vi "NumIntegrate_Rkf45_Ax_Bu_K.vi"(5 "A":T1, 6 "MaxError":dbl=1e-06, 7 "B":T1, 8 "dT_Seconds":dbl, 9 "K":T1, 10 "U":T1, 11 "X":T1) -> (1 "IterationCount":i32, 3 "Return X":T1)   [LabVIEW 2019, in "Trajectory_Library.lvlib"]
doc: "Creates a new LINEAR SYSTEM data cluster with the specified values. \n\n\nInputs: \n - XXX -- XXX.\n\nOutputs:\n - XXX -- XXX."
uses:
  Trajectory_Library.lvlib
  <vilib>/Analysis/Matrix/Datatypes/RealMatrix.ctl
  <vilib>/Analysis/Matrix/NI_Matrix.lvlib
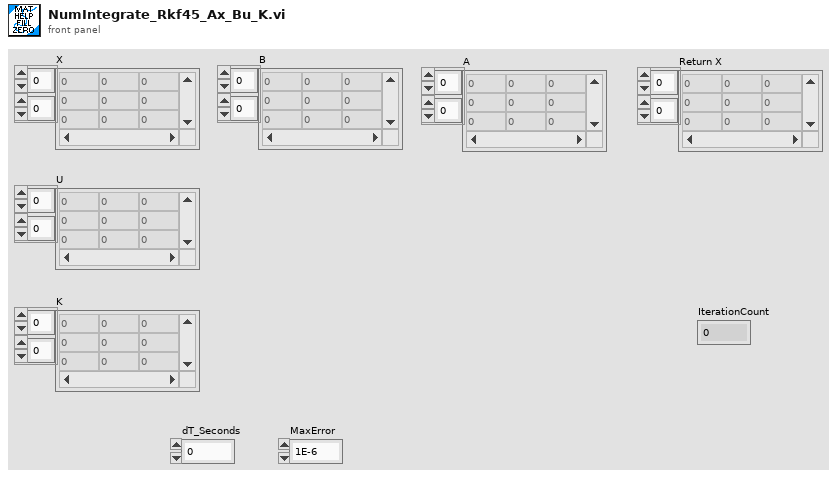
[diagram p1: front panel]
types:
  T1 = typedef "NI_Matrix.lvlib/RealMatrix.ctl" = dbl[][]
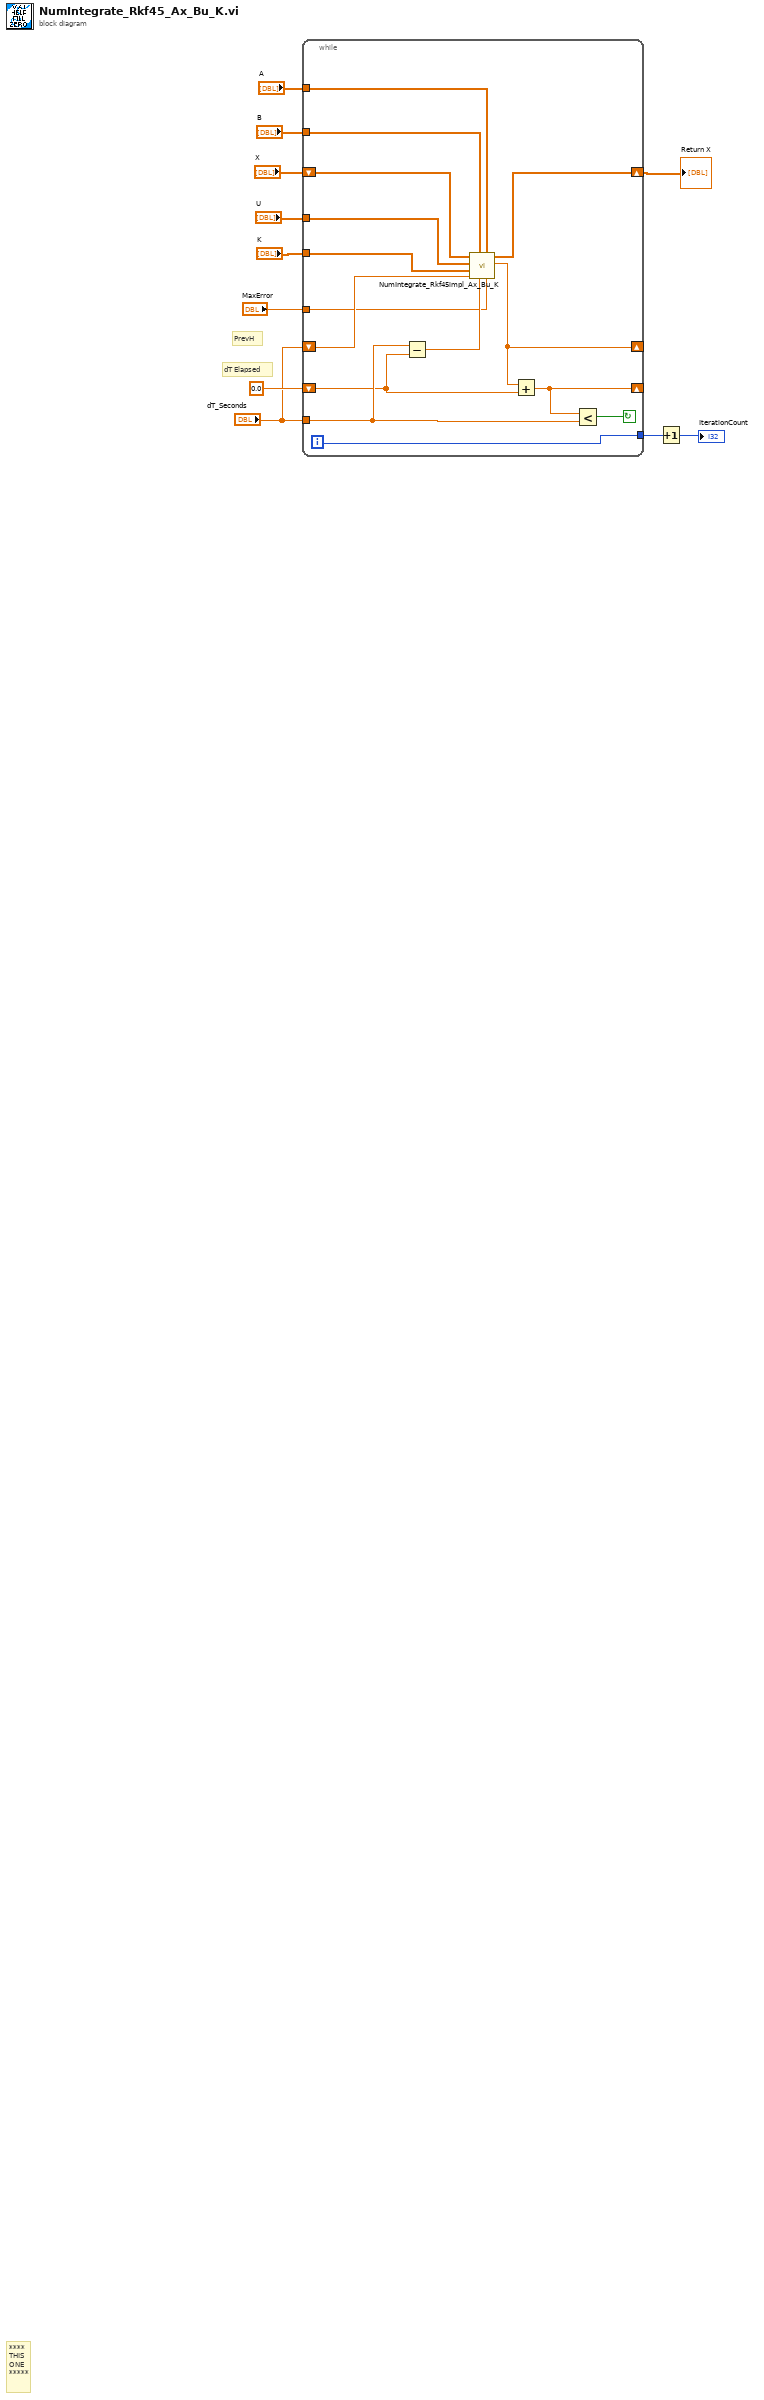
[diagram p0: block diagram]
diagram:
  # "PrevH"
  # "dT Elapsed"
  # "****\nTHIS\nONE\n*****"
  n1 = while {
    shift-right: [w15] -> _
    shift-left: 0.0 -> [w14]
    tunnel: "dT_Seconds" -> [w18]
    shift-right: [w13] -> _
    shift-left: "dT_Seconds" -> [w19]
    tunnel: "A" -> [w25]
    tunnel: "B" -> [w24]
    shift-right: [w22] -> w4
    shift-left: "X" -> [w23]
    tunnel: "U" -> [w21]
    tunnel: "K" -> [w20]
    tunnel: "MaxError" -> [w16]
    tunnel: [w12] -> w1
    i -> [w12]
    stop <- w26 continue-if-true
    n2 = Subtract(x=w18, y=w14) -> (x-y=w17:dbl)
    n3 = call "NumIntegrate_Rkf45impl_Ax_Bu_K.vi"("MaxTruncError"=w16, "A"=w25, "dT_Remaining"=w17, "B"=w24, "InitialH"=w19, "K"=w20, "U"=w21, "X"=w23) -> ("H"=w13:dbl, "NewX"=w22:T1)  [unwired: 1 in, 1 out]
    n4 = Add(x=w13, y=w14) -> (x+y=w15:dbl)
    n5 = Less?(x=w15, y=w18) -> (x < y?=w26:bool)
  }
  "Return X" <- w4
  n6 = Increment(x=w1) -> (x+1=→"IterationCount":i32)
